vi "TestFlipper.vi"() -> ()   [LabVIEW 2020]
uses:
  C:/Program Files (x86)/Thorlabs/Kinesis/Thorlabs.MotionControl.FilterFlipperCLI.dll
  Program Files (x86)/Thorlabs/Kinesis/Thorlabs.MotionControl.FilterFlipperCLI.dll
  C:/Program Files (x86)/Thorlabs/Kinesis/Thorlabs.MotionControl.DeviceManagerCLI.dll
  Program Files (x86)/Thorlabs/Kinesis/Thorlabs.MotionControl.DeviceManagerCLI.dll
panel:
  in  "Postion":enum32{"NA", "Position1", "Position2"}(ring)
  in  "GET":bool
  in  "SET":bool
  in  "position":u32
  in  "INIT":bool
  out "Status array":bool[](array[boolean])
  in  "OK":bool
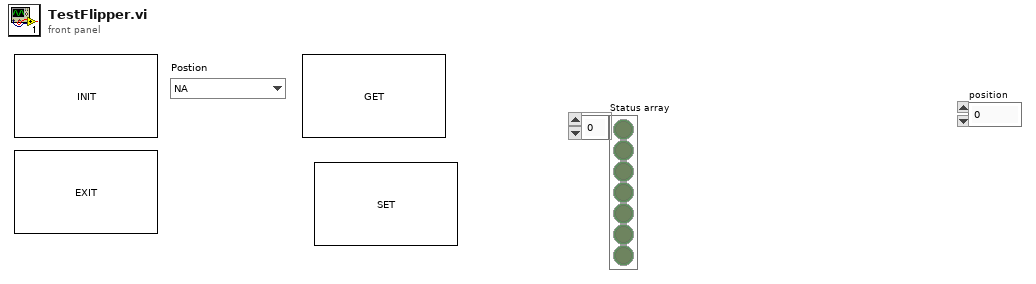
[diagram p1: front panel]
types:
  T1 = enum32{"Invalid", "Standard", "Closed", "Hidden", "Minimized", "Maximized"}
  T2 = enum32{"invalid app kind", "Development System", "Run Time System", "Student Edition", "Embedded LabVIEW", "Evaluation", "Custom"}
  T3 = cluster{"Core":cluster{"Current VI Reference":refnum<vi>, "Close Panel on Exit?":bool}, "Flipper":refnum<k24>, "Device":refnum<k24>}
  T4 = cluster{"Current VI Reference":refnum<vi>, "Close Panel on Exit?":bool}
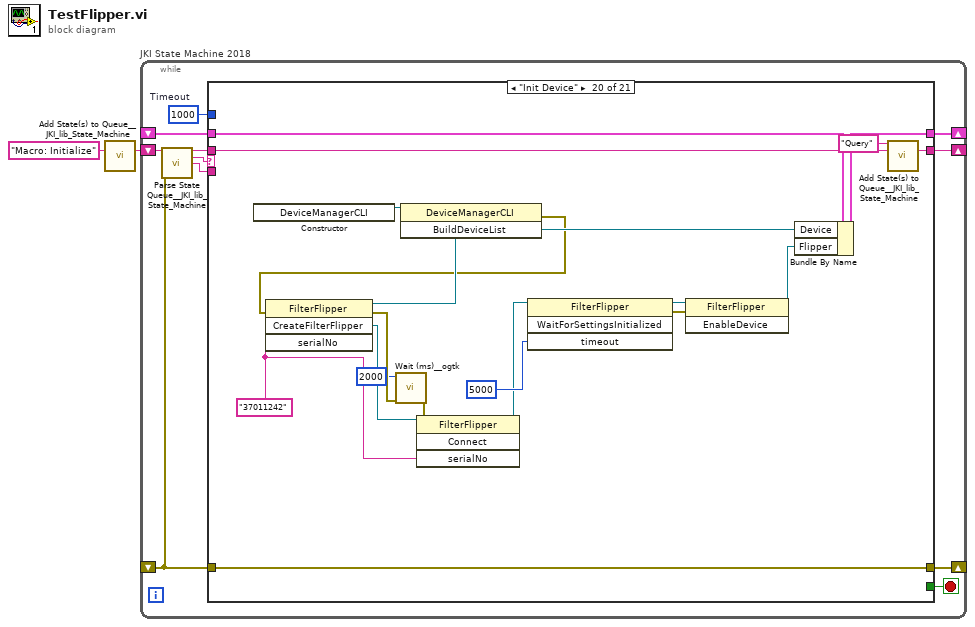
[diagram p0: block diagram]
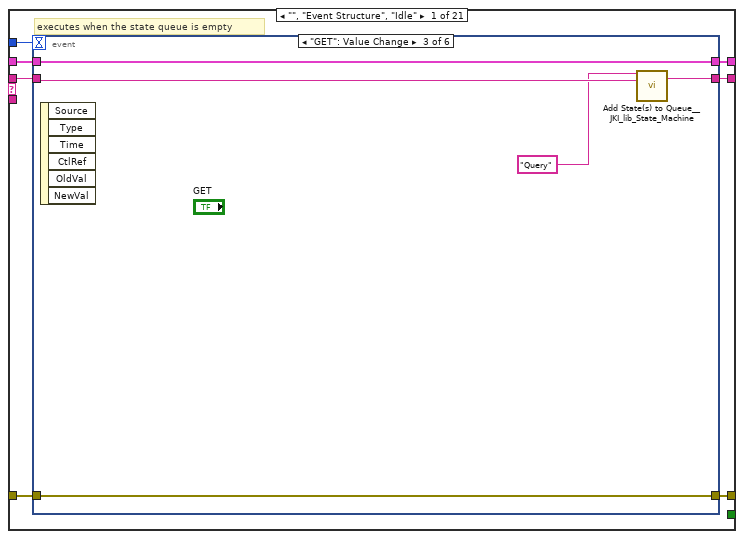
[diagram p2: hidden frame]
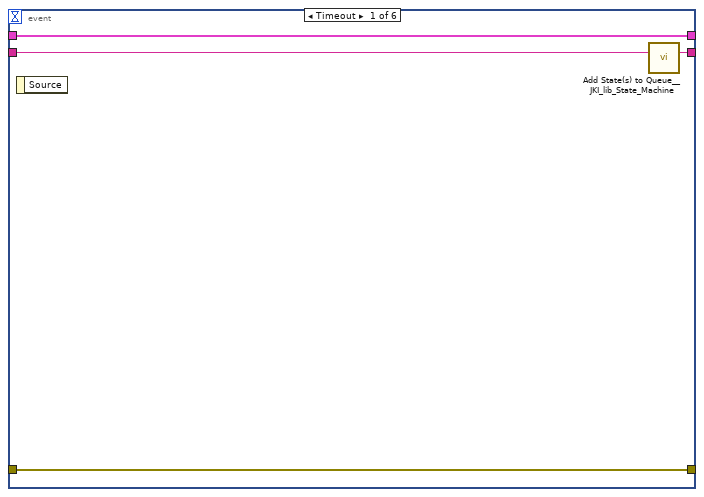
[diagram p3: hidden frame]
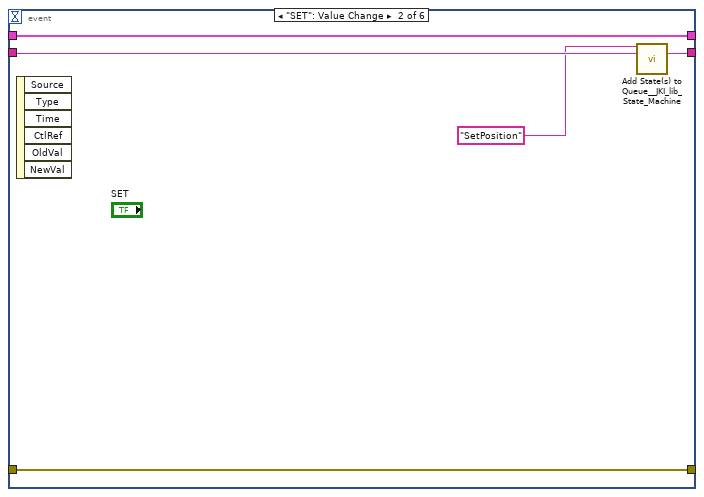
[diagram p4: hidden frame]
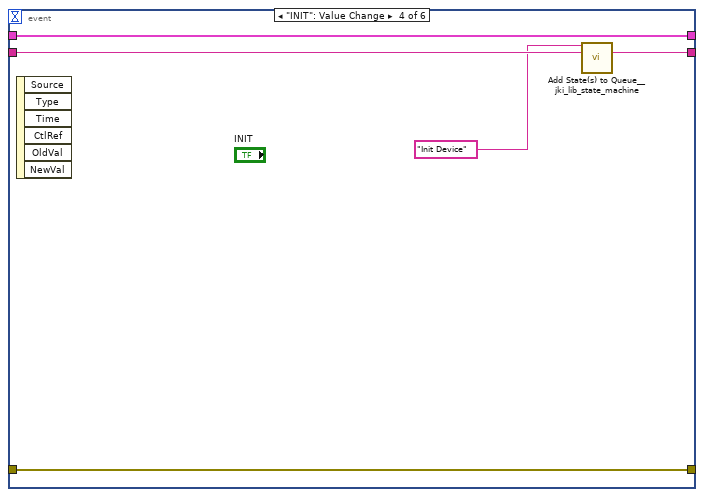
[diagram p5: hidden frame]
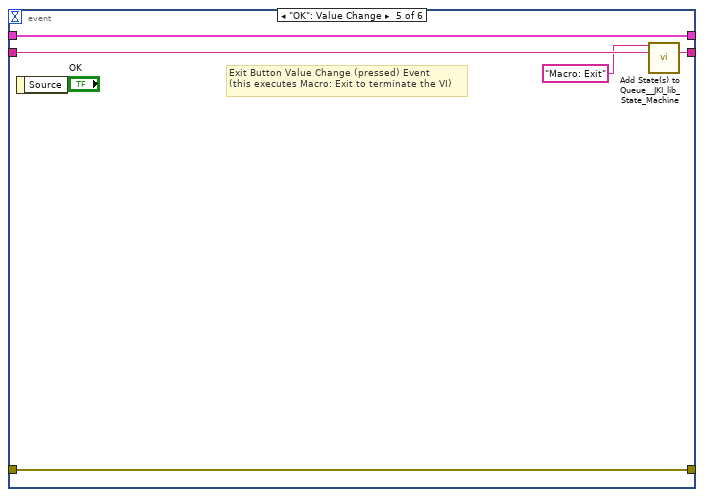
[diagram p6: hidden frame]
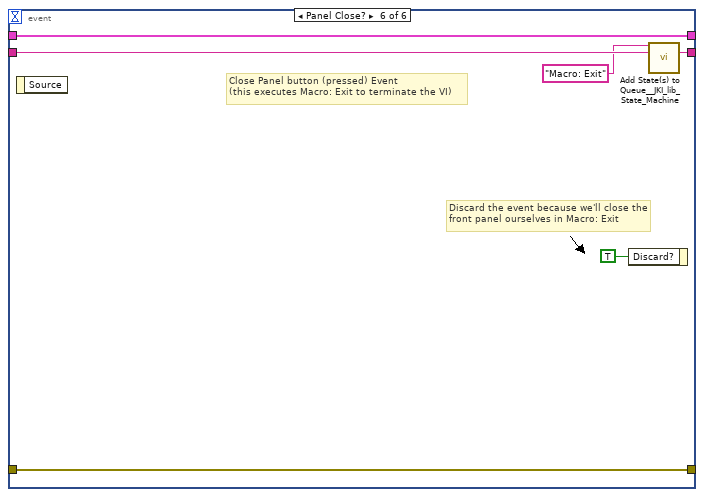
[diagram p7: hidden frame]
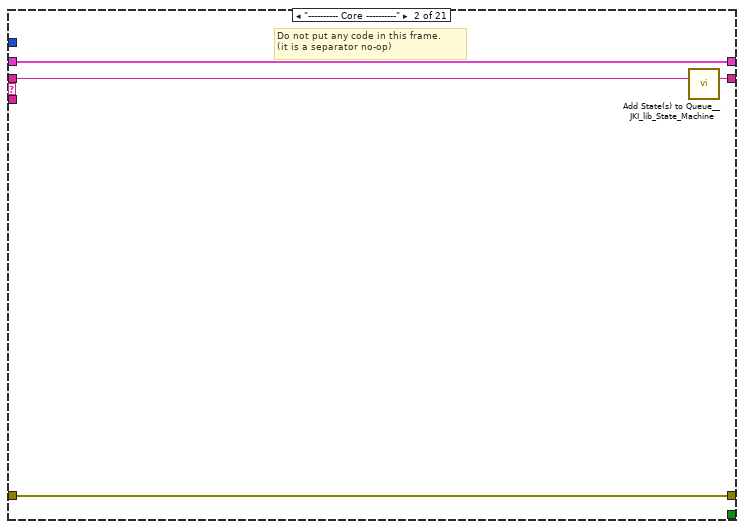
[diagram p8: hidden frame]
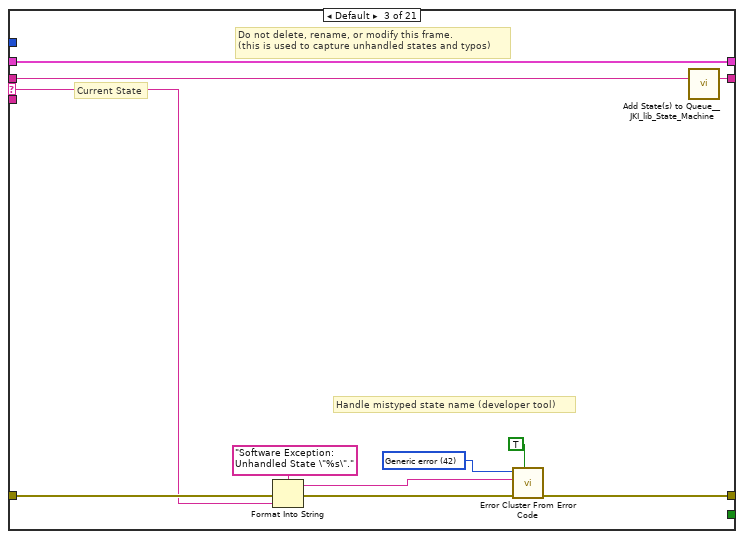
[diagram p9: hidden frame]
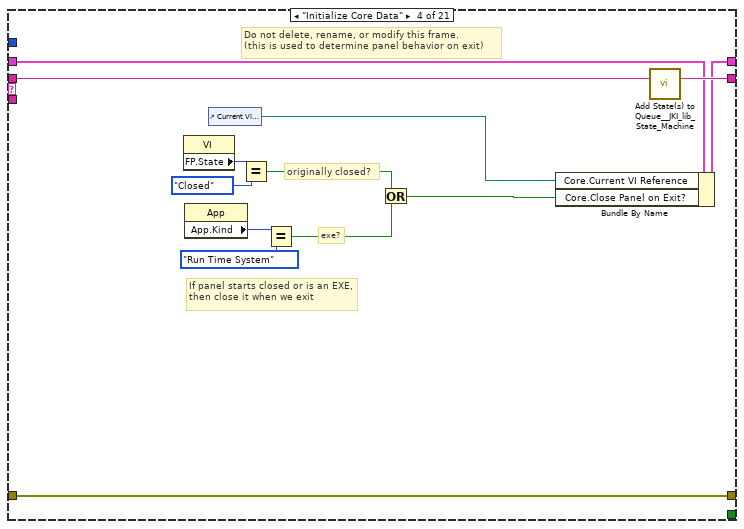
[diagram p10: hidden frame]
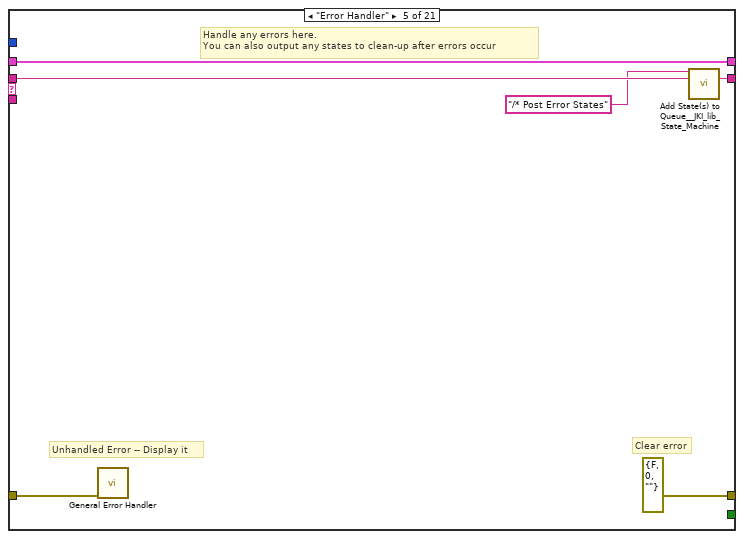
[diagram p11: hidden frame]
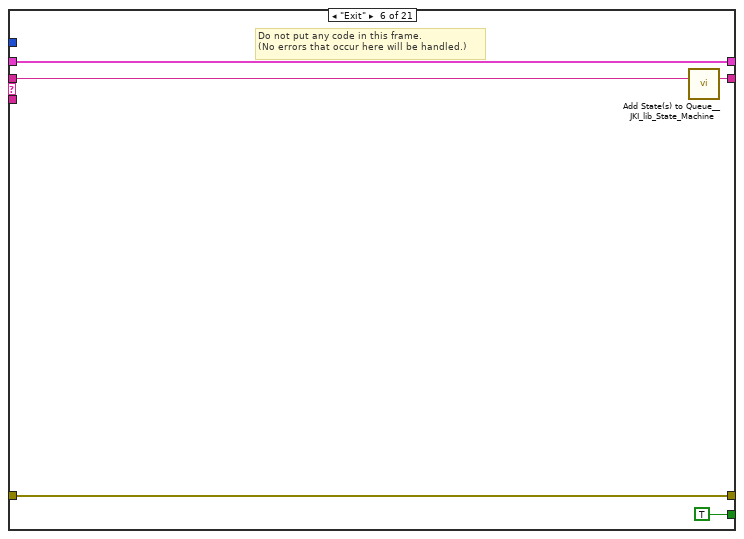
[diagram p12: hidden frame]
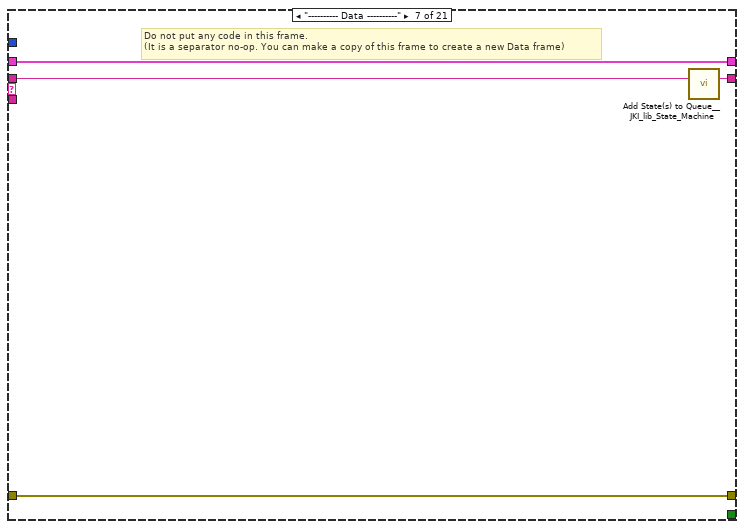
[diagram p13: hidden frame]
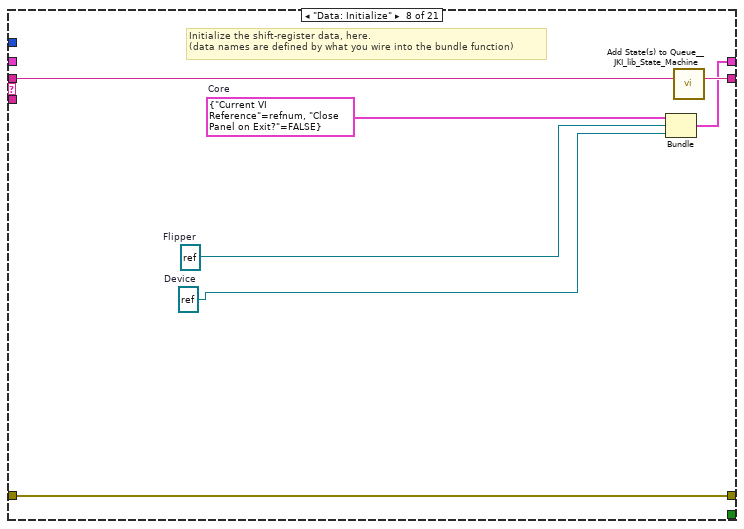
[diagram p14: hidden frame]
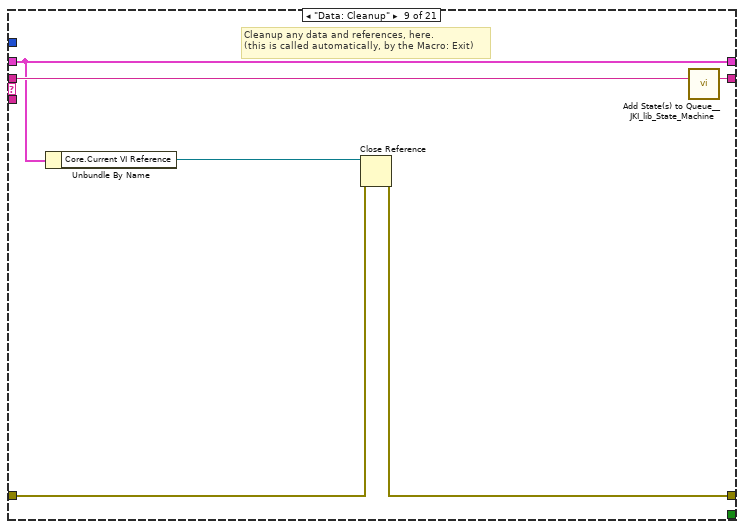
[diagram p15: hidden frame]
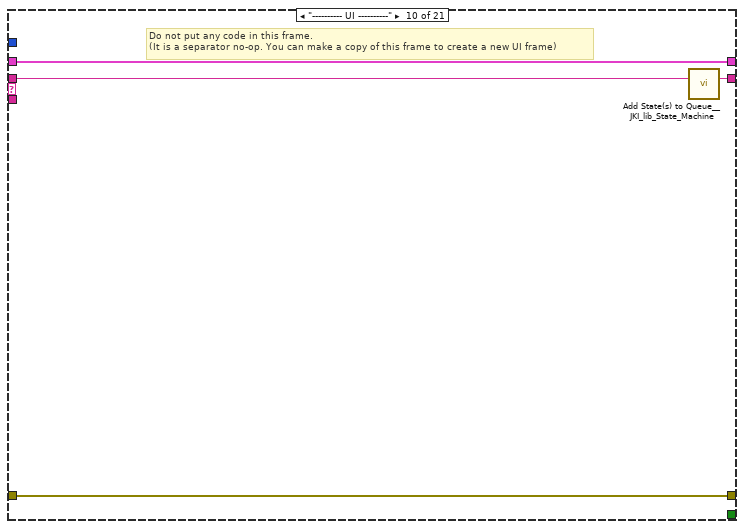
[diagram p16: hidden frame]
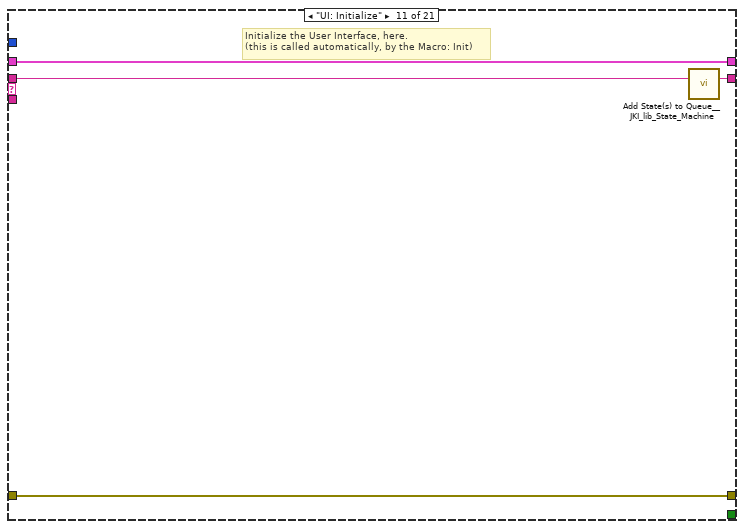
[diagram p17: hidden frame]
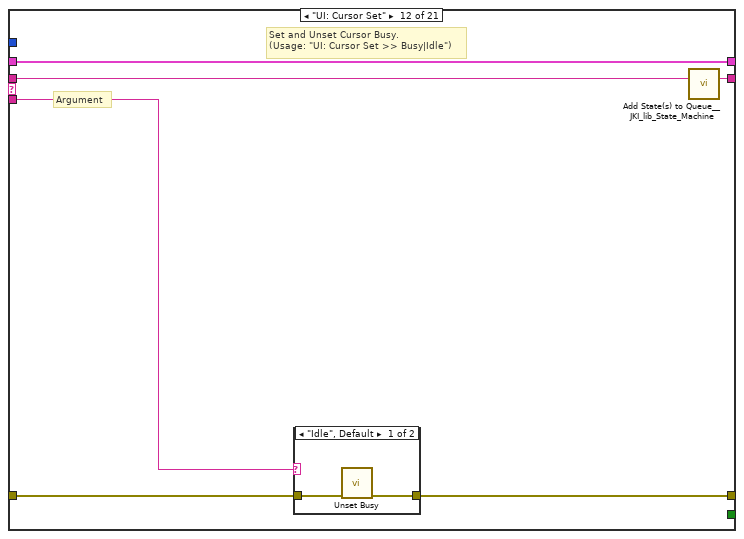
[diagram p18: hidden frame]
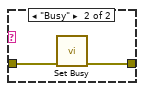
[diagram p19: hidden frame]
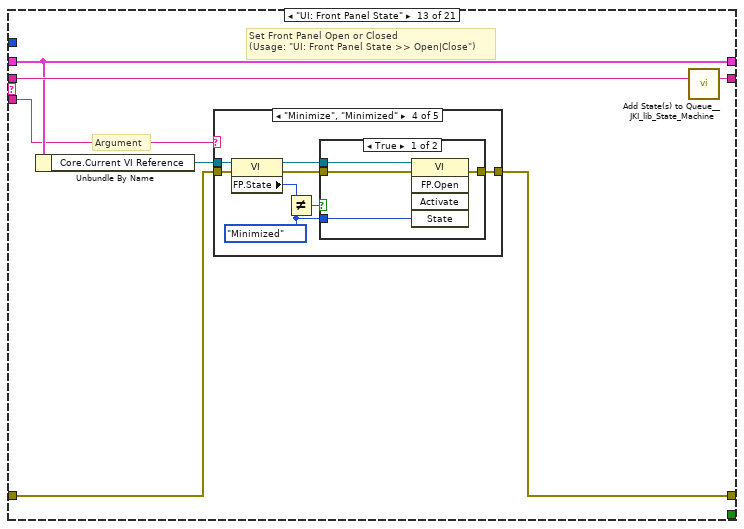
[diagram p20: hidden frame]
diagram:
  n1 = call <vilib>:"Add State(s) to Queue__JKI_lib_State_Machine.vi"("State(s) in (\"\")"="Macro: Initialize") -> ("States Out"=w2:string)  [unwired: 14 in]
  n2 = while "JKI State Machine 2018" {
    shift-right: [w6] -> _
    shift-left: _ -> [w5]
    shift-right: [w9] -> _
    shift-left: _ -> [w3]
    shift-right: [w8] -> _
    shift-left: w2 -> [w10]
    stop <- w7 stop-if-true
    w4 = 1000  # Timeout
    n3 = call <vilib>:"Parse State Queue__JKI_lib_State_Machine.vi"("State Queue"=w10, "Error In (no error)"=w3) -> ("Remaining States"=w12:string, "Current State"=w13:string, "Arguments"=w11:string)  [unwired: 11 in]
    n4 = case shown="\"Init Device\"" w13 {
      selector: w13 -> [_ _ w55 _ _ _ _ _ _ _ _ _ _ _ _ _ _ _ _ _ _]
      tunnel: w12 -> [w20 w54 w59 w78 w84 w89 w93 w100 w106 w110 w114 w120 w131 w200 w205 w215 w219 w235 w247 w266 w281]
      tunnel: w11 -> [_ _ _ _ _ _ _ _ _ _ _ w115 w125 _ _ _ _ _ _ _ _]
      tunnel: w5 -> [w18 w51 w57 w71 w81 w87 w90 _ w101 w107 w112 w118 w127 w197 w202 w212 w216 w233 w241 w263 w271]
      tunnel: [w17 w52 w61 w75 errorcluster {"status"=FALSE, "code"=0, "source"=""} ("error out") w86 w91 w97 w102 w108 w111 w116 w128 w198 w203 w213 w217 w221 w245 w264 w279] -> w9
      tunnel: w3 -> [w16 w52 w60 w75 w80 w86 w91 w97 w103 w108 w111 w117 w129 w198 w203 w213 w217 w229 w245 w264 w279]
      tunnel: [w19 w53 w58 w77 w83 w88 w92 w99 w105 w109 w113 w119 w130 w199 w204 w214 w218 w234 w246 w265 w280] -> w8
      tunnel: [_ _ _ _ _ TRUE _ _ _ _ _ _ _ _ _ _ _ _ _ _ _] -> w7
      tunnel: [w15 w51 w57 w76 w81 w87 w90 w98 w101 w107 w112 w118 w127 w197 w202 w212 w216 w230 w241 w259 w270] -> w6
      tunnel: w4 -> [w14 _ _ _ _ _ _ _ _ _ _ _ _ _ _ _ _ _ _ _ _]
      frame "", "Event Structure", "Idle" {
        # "executes when the state queue is empty"
        n5 = event shown="[2] \"GET\": Value Change" {
          selector: _ -> [_ _ _ _ _ _]
          dyn-events: _ -> [_ _ _ _ _ _]
          timeout: w14 -> [_ _ _ _ _ _]
          tunnel: w20 -> [w24 w26 w32 w37 w44 w50]
          tunnel: [w23 w27 w33 w36 w43 w49] -> w19
          tunnel: w18 -> [w21 w29 w34 w39 w41 w47]
          tunnel: [w22 w28 w30 w38 w42 w48] -> w17
          tunnel: w16 -> [w22 w28 w30 w38 w42 w48]
          tunnel: [w21 w29 w34 w39 w41 w47] -> w15
          event Timeout {
            n6 = event-data() -> ()  [unwired: 1 in, 1 out]
            n7 = call <vilib>:"Add State(s) to Queue__JKI_lib_State_Machine.vi"("State(s) in (\"\")"=w24) -> ("States Out"=w23:string)  [unwired: 14 in]
          }
          event "SET": Value Change {
            n8 = event-data() -> ()  [unwired: 1 in, 6 out]
            n9 = call <vilib>:"Add State(s) to Queue__JKI_lib_State_Machine.vi"("State(s) in Front (\"\")"="SetPosition" ("State(s) in Front (\"\")"), "State(s) in (\"\")"=w26) -> ("States Out"=w27:string)  [unwired: 13 in]
          }
          event "GET": Value Change {
            n10 = event-data() -> ()  [unwired: 1 in, 6 out]
            n11 = call <vilib>:"Add State(s) to Queue__JKI_lib_State_Machine.vi"("State(s) in Front (\"\")"="Query" ("State(s) in Front (\"\")"), "State(s) in (\"\")"=w32) -> ("States Out"=w33:string)  [unwired: 13 in]
          }
          event "INIT": Value Change {
            n12 = event-data() -> ()  [unwired: 1 in, 6 out]
            n13 = call <vilib>:"Add State(s) to Queue__jki_lib_state_machine.vi"("State(s) in Front (\"\")"="Init Device" ("State(s) in Front (\"\")"), "State(s) in (\"\")"=w37) -> ("States Out"=w36:string)  [unwired: 13 in]
          }
          event "OK": Value Change {
            # "Exit Button Value Change (pressed) Event\n(this executes Macro: Exit to terminate the VI)"
            n14 = event-data() -> ()  [unwired: 1 in, 1 out]
            n15 = call <vilib>:"Add State(s) to Queue__JKI_lib_State_Machine.vi"("State(s) in Front (\"\")"="Macro: Exit", "State(s) in (\"\")"=w44) -> ("States Out"=w43:string)  [unwired: 13 in]
          }
          event Panel Close? {
            # "Discard the event because we'll close the front panel ourselves in Macro: Exit"
            # "Close Panel button (pressed) Event\n(this executes Macro: Exit to terminate the VI)"
            n16 = event-data() -> ()  [unwired: 1 in, 1 out]
            n17 = event-data("Discard?"=TRUE) -> ()  [unwired: 1 in, 1 out]
            n18 = call <vilib>:"Add State(s) to Queue__JKI_lib_State_Machine.vi"("State(s) in Front (\"\")"="Macro: Exit", "State(s) in (\"\")"=w50) -> ("States Out"=w49:string)  [unwired: 13 in]
          }
        }
      }
      frame "---------- Core ----------" {
        # "Do not put any code in this frame.\n(it is a separator no-op)"
        n19 = call <vilib>:"Add State(s) to Queue__JKI_lib_State_Machine.vi"("State(s) in (\"\")"=w54) -> ("States Out"=w53:string)  [unwired: 14 in]
      }
      frame Default {
        w64 = 42 items=["No error", "Argument error", "Memory is full", "Out of zone", "End of file", "File already open", "Generic file I/O error", "File not found", "File permission error", "Disk is full", "Duplicate path", "Too many files open", "System feature not enabled", "Resource file not found", "Cannot add resource", "Resource not found", "Image not found", "Image memory error", "Pen does not exist", "Config type invalid", "Config token not found", "Config parse error", "Config memory error", "Bad external code format", "Bad external code offset", "External code not present", "Null window", "Destroy window error", "Null menu", "Print aborted", "Bad print record", "Print driver error", "Windows error during printing", "Memory error during printing", "Print dialog error", "Generic print error", "Invalid device refnum", "Device not found", "Device parameter error", "Device unit error", "Cannot open device", "Device call aborted", "Generic error", "Cancelled by user", "Object ID too low", "Object ID too high", "Object not in heap", "Unknown heap", "Unknown object (invalid DefProc)", "Unknown object (DefProc not in table)", "Message out of range", "Invalid (null) method", "Unknown message", "Manager call not supported", "Bad address", "Network operation in progress", "Network operation timed out", "Connection is busy", "Network attribute not supported", "Network error", "Address in use", "System out of memory", "Connection aborted", "Connection refused", "Not connected", "Already connected", "Connection closed", "Initialization error (interapplication manager)", "Bad occurrence", "Wait on unbound occurrence handler", "Occurrence queue overflow", "Datalog type conflict", "Unused", "Unrecognized type (interapplication manager)", "Memory corrupt", "Failed to make temporary DLL", "Old CIN version", "Drag socket not found", "Failed to load drop-object", "Failed to register OLE object", "Failed to release OLE object", "Format specifier type mismatch", "Unknown format specifier", "Too few format specifiers", "Too many format specifiers", "Scan failed", "Newer CIN version", "Error converting to variant", "Runtime menu error", "Password tampered", "Variant attribute not found", "Incompatible variant data type", "Event data is not available", "Event Store is not present", "Occurrence is not found", "Event Queue is not created", "Event info is not available", "Refnum passed is NULL", "Error retrieving Class GUID", "Error retrieving CoClass GUID", "Error retrieving TypeLib GUID.", "Bad built application magic bytes.", "Specific driver is different from the specific driver associated with the Logical Name.", "There is no session opened to the class driver.", "Max Error", "MAX - Error with config objects", "MAX - Error loading configuration", "MAX - Group not supported"]
        # "Current State"
        # "Do not delete, rename, or modify this frame.\n(this is used to capture unhandled states and typos)"
        # "Handle mistyped state name (developer tool)"
        n20 = Format Into String(format string="Software Exception: Unhandled State \"%s\"." ("message"), error in=w60, w55) -> (resulting string=w63:string, error out=w62:errorcluster)  [unwired: 1 in]
        n21 = call <vilib>:"Error Cluster From Error Code.vi"("show call chain? (False)"=TRUE, "error in (no error)"=w62, "error message (\"\")"=w63, "error code (0)"=w64) -> ("error out"=w61:errorcluster)  [unwired: 5 in]
        n22 = call <vilib>:"Add State(s) to Queue__JKI_lib_State_Machine.vi"("State(s) in (\"\")"=w59) -> ("States Out"=w58:string)  [unwired: 14 in]
      }
      frame "Initialize Core Data" {
        # "Do not delete, rename, or modify this frame.\n(this is used to determine panel behavior on exit)"
        # "originally closed?"
        # "exe?"
        # "If panel starts closed or is an EXE, then close it when we exit"
        n23 = property class="VI"() -> ("FP.State"=w68:T1)  [unwired: 2 in, 2 out]
        n24 = property class="App"() -> ("App.Kind"=w74:T2)  [unwired: 2 in, 2 out]
        n25 = control-ref of="Current VI Reference"() -> (w69:refnum<vi>)
        n26 = Equal?(x=w68, y=T1."Closed" ("Front Panel Window:State")) -> (x = y?=w66:bool)
        n27 = Equal?(x=w74, y=T2."Run Time System" ("Application:Kind")) -> (x = y?=w72:bool)
        n28 = Or(x=w66, y=w72) -> (x .or. y?=w70:bool)
        n29 = Bundle By Name(cluster=w71, "Core.Current VI Reference"=w69, "Core.Close Panel on Exit?"=w70) -> (w76:T3)
        n30 = call <vilib>:"Add State(s) to Queue__JKI_lib_State_Machine.vi"("State(s) in (\"\")"=w78) -> ("States Out"=w77:string)  [unwired: 14 in]
      }
      frame "Error Handler" {
        # "Unhandled Error -- Display it"
        # "Handle any errors here.\nYou can also output any states to clean-up after errors occur"
        # "Clear error"
        n31 = call <vilib>:"General Error Handler.vi"("error in (no error)"=w80) -> ()  [unwired: 10 in, 5 out]
        n32 = call <vilib>:"Add State(s) to Queue__JKI_lib_State_Machine.vi"("State(s) in Front (\"\")"="/* Post Error States", "State(s) in (\"\")"=w84) -> ("States Out"=w83:string)  [unwired: 13 in]
      }
      frame "Exit" {
        # "Do not put any code in this frame.\n(No errors that occur here will be handled.)"
        n33 = call <vilib>:"Add State(s) to Queue__JKI_lib_State_Machine.vi"("State(s) in (\"\")"=w89) -> ("States Out"=w88:string)  [unwired: 14 in]
      }
      frame "---------- Data ----------" {
        # "Do not put any code in this frame.\n(It is a separator no-op. You can make a copy of this frame to create a new Data frame)"
        n34 = call <vilib>:"Add State(s) to Queue__JKI_lib_State_Machine.vi"("State(s) in (\"\")"=w93) -> ("States Out"=w92:string)  [unwired: 14 in]
      }
      frame "Data: Initialize" {
        w94 = refnum<k24> refnum  # Device
        w95 = refnum<k24> refnum  # Flipper
        w96 = T4 {"Current VI Reference"=refnum, "Close Panel on Exit?"=FALSE}  # Core
        # "Initialize the shift-register data, here.\n(data names are defined by what you wire into the bundle function)"
        n35 = Bundle("Core"=w96, "Flipper"=w95, "Device"=w94) -> (w98:T3)  [unwired: 1 in]
        n36 = call <vilib>:"Add State(s) to Queue__JKI_lib_State_Machine.vi"("State(s) in (\"\")"=w100) -> ("States Out"=w99:string)  [unwired: 14 in]
      }
      frame "Data: Cleanup" {
        # "Cleanup any data and references, here.\n(this is called automatically, by the Macro: Exit)"
        n37 = Unbundle By Name(w101) -> ("Core.Current VI Reference"=w104:refnum<vi>)
        n38 = Close Reference(reference=w104, error in (no error)=w103) -> (error out=w102:errorcluster)
        n39 = call <vilib>:"Add State(s) to Queue__JKI_lib_State_Machine.vi"("State(s) in (\"\")"=w106) -> ("States Out"=w105:string)  [unwired: 14 in]
      }
      frame "---------- UI ----------" {
        # "Do not put any code in this frame.\n(It is a separator no-op. You can make a copy of this frame to create a new UI frame)"
        n40 = call <vilib>:"Add State(s) to Queue__JKI_lib_State_Machine.vi"("State(s) in (\"\")"=w110) -> ("States Out"=w109:string)  [unwired: 14 in]
      }
      frame "UI: Initialize" {
        # "Initialize the User Interface, here.\n(this is called automatically, by the Macro: Init)"
        n41 = call <vilib>:"Add State(s) to Queue__JKI_lib_State_Machine.vi"("State(s) in (\"\")"=w114) -> ("States Out"=w113:string)  [unwired: 14 in]
      }
      frame "UI: Cursor Set" {
        # "Argument"
        # "Set and Unset Cursor Busy.\n(Usage: \"UI: Cursor Set >> Busy|Idle\")"
        n42 = case shown="\"Idle\", Default" w115 {
          tunnel: w117 -> [w122 w124]
          tunnel: [w121 w123] -> w116
          frame "Idle", Default {
            n43 = call <vilib>:"Unset Busy.vi"("error in (no error)"=w122) -> ("error out"=w121:errorcluster)  [unwired: 10 in]
          }
          frame "Busy" {
            n44 = call <vilib>:"Set Busy.vi"("error in (no error)"=w124) -> ("error out"=w123:errorcluster)  [unwired: 9 in, 1 out]
          }
        }
        n45 = call <vilib>:"Add State(s) to Queue__JKI_lib_State_Machine.vi"("State(s) in (\"\")"=w120) -> ("States Out"=w119:string)  [unwired: 14 in]
      }
      frame "UI: Front Panel State" {
        # "Argument"
        # "Set Front Panel Open or Closed\n(Usage: \"UI: Front Panel State >> Open|Close\")"
        n46 = Unbundle By Name(w127) -> ("Core.Current VI Reference"=w126:refnum<vi>)
        n47 = case shown="\"Minimize\", \"Minimized\"" w125 {
          tunnel: w129 -> [w137 w152 w163 w176 w189]
          tunnel: [w139 w153 w165 w178 w191] -> w128
          tunnel: w126 -> [w138 w150 w164 w177 w190]
          frame "Open", "Standard", Default {
            w132 = T1."Standard" ("State")
            n48 = property class="VI"(reference=w138, error in=w137) -> (reference out=w135:refnum<vi>, error out=w136:errorcluster, "FP.State"=w134:T1)
            n49 = Not Equal?(x=w134, y=w132) -> (x != y?=w133:bool)
            n50 = case shown="True" w133 {
              tunnel: [w143 w145] -> w139
              tunnel: w136 -> [w142 w145]
              tunnel: w135 -> [w141 _]
              tunnel: w132 -> [w140 _]
              frame True {
                n51 = invoke class="VI" method="FP.Open"(reference=w141, error in=w142, "Activate"=TRUE, "State"=w140) -> (error out=w143:errorcluster)  [unwired: 1 in, 4 out]
              }
              frame False {
              }
            }
          }
          frame "Close", "Closed" {
            n52 = property class="VI"(reference=w150, error in=w152) -> (reference out=w149:refnum<vi>, error out=w151:errorcluster, "FP.State"=w147:T1)
            n53 = Not Equal?(x=w147, y=T1."Closed" ("Front Panel Window:State")) -> (x != y?=w146:bool)
            n54 = case shown="True" w146 {
              tunnel: [w154 w157] -> w153
              tunnel: w151 -> [w154 w156]
              tunnel: w149 -> [_ w155]
              frame False {
              }
              frame True {
                n55 = invoke class="VI" method="FP.Close"(reference=w155, error in=w156) -> (error out=w157:errorcluster)  [unwired: 1 in, 2 out]
              }
            }
          }
          frame "Hidden", "Hide" {
            w158 = T1."Hidden" ("State")
            n56 = property class="VI"(reference=w164, error in=w163) -> (reference out=w161:refnum<vi>, error out=w162:errorcluster, "FP.State"=w160:T1)
            n57 = Not Equal?(x=w160, y=w158) -> (x != y?=w159:bool)
            n58 = case shown="True" w159 {
              tunnel: [w169 w170] -> w165
              tunnel: w162 -> [w168 w170]
              tunnel: w161 -> [w167 _]
              tunnel: w158 -> [w166 _]
              frame True {
                n59 = invoke class="VI" method="FP.Open"(reference=w167, error in=w168, "State"=w166) -> (error out=w169:errorcluster)  [unwired: 2 in, 4 out]
              }
              frame False {
              }
            }
          }
          frame "Minimize", "Minimized" {
            w171 = T1."Minimized" ("State")
            n60 = property class="VI"(reference=w177, error in=w176) -> (reference out=w174:refnum<vi>, error out=w175:errorcluster, "FP.State"=w173:T1)
            n61 = Not Equal?(x=w173, y=w171) -> (x != y?=w172:bool)
            n62 = case shown="True" w172 {
              tunnel: [w182 w183] -> w178
              tunnel: w175 -> [w181 w183]
              tunnel: w174 -> [w180 _]
              tunnel: w171 -> [w179 _]
              frame True {
                n63 = invoke class="VI" method="FP.Open"(reference=w180, error in=w181, "State"=w179) -> (error out=w182:errorcluster)  [unwired: 2 in, 4 out]
              }
              frame False {
              }
            }
          }
          frame "Maximize", "Maximized" {
            w184 = T1."Maximized" ("State")
            n64 = property class="VI"(reference=w190, error in=w189) -> (reference out=w187:refnum<vi>, error out=w188:errorcluster, "FP.State"=w186:T1)
            n65 = Not Equal?(x=w186, y=w184) -> (x != y?=w185:bool)
            n66 = case shown="True" w185 {
              tunnel: [w195 w196] -> w191
              tunnel: w188 -> [w194 w196]
              tunnel: w187 -> [w193 _]
              tunnel: w184 -> [w192 _]
              frame True {
                n67 = invoke class="VI" method="FP.Open"(reference=w193, error in=w194, "State"=w192) -> (error out=w195:errorcluster)  [unwired: 2 in, 4 out]
              }
              frame False {
              }
            }
          }
        }
        n68 = call <vilib>:"Add State(s) to Queue__JKI_lib_State_Machine.vi"("State(s) in (\"\")"=w131) -> ("States Out"=w130:string)  [unwired: 14 in]
      }
      frame "---------- Macro ----------" {
        # "Do not put any code in this frame.\n(It is a separator no-op. You can make a copy of this frame to create a new Macro frame)"
        n69 = call <vilib>:"Add State(s) to Queue__JKI_lib_State_Machine.vi"("State(s) in (\"\")"=w200) -> ("States Out"=w199:string)  [unwired: 14 in]
      }
      frame "Macro: Initialize" {
        w201 = "Data: Initialize\nInitialize Core Data\nUI: Initialize\nUI: Front Panel State >> Open"  # Data: Initialize Initialize Core Data UI: Initialize UI: Front Panel State >> Open
        # "Initialization Macro\n(This is called once, when the VI starts)"
        n70 = call <vilib>:"Add State(s) to Queue__JKI_lib_State_Machine.vi"("State(s) in Front (\"\")"=w201, "State(s) in (\"\")"=w205) -> ("States Out"=w204:string)  [unwired: 13 in]
      }
      frame "Macro: Exit" {
        # "Exit Macro\n(This is called once, when the VI exits)"
        n71 = Unbundle By Name(w212) -> ("Core.Close Panel on Exit?"=w211:bool)
        n72 = Select(t="UI: Front Panel State >> Close", s=w211, f="") -> (s? t:f=w208:string)
        n73 = call <vilib>:"Add State(s) to Queue__JKI_lib_State_Machine.vi"("State(s) in (\"\")"=w208, "State(s) at Back (\"\")"="DIsconnnect\nData: Cleanup\nExit") -> ("States Out"=w206:string)  [unwired: 13 in]
        n74 = call <vilib>:"Add State(s) to Queue__JKI_lib_State_Machine.vi"("State(s) in Front (\"\")"=w206, "State(s) in (\"\")"=w215) -> ("States Out"=w214:string)  [unwired: 13 in]
      }
      frame "---------- New Category ----------" {
        # "Template Separator\n(You can make a copy of, or modify, this frame)"
        n75 = call <vilib>:"Add State(s) to Queue__JKI_lib_State_Machine.vi"("State(s) in (\"\")"=w219) -> ("States Out"=w218:string)  [unwired: 14 in]
      }
      frame "SetPosition" {
        n76 = Unbundle By Name(w233) -> ("Flipper"=w228:refnum<k24>)
        n77 = invoke class="FilterFlipper" method="ClearDeviceExceptions"(reference=w228) -> (reference out=w227:refnum<k24>)  [unwired: 2 in, 2 out]
        n78 = invoke class="FilterFlipper" method="SetPosition"(reference=w227, error in=w229, "position"="Postion", "waitTimeout"=2000) -> (reference out=w224:refnum<k24>, error out=w226:errorcluster)  [unwired: 1 in, 3 out]
        n79 = call <userlib>:"Wait (ms)__ogtk.vi"("error in (no error)"=w226, "milliseconds to wait"=u32 50) -> ("error out"=w222:errorcluster)  [unwired: 8 in, 1 out]
        n80 = Unbundle By Name(w222) -> ("code"=w223:i32)
        n81 = case shown="0, Default" w223 {
          tunnel: [w236 errorcluster {"status"=FALSE, "code"=0, "source"=""} ("error out")] -> w221
          tunnel: w222 -> [w236 _]
          frame 0, Default {
          }
          frame 1172 {
          }
        }
        n82 = Bundle By Name(cluster=w233, "Flipper"=w224) -> (w230:T3)
        n83 = call <vilib>:"Add State(s) to Queue__JKI_lib_State_Machine.vi"("State(s) in Front (\"\")"="Query" ("State(s) in Front (\"\")"), "State(s) in (\"\")"=w235) -> ("States Out"=w234:string)  [unwired: 13 in]
      }
      frame "DIsconnnect" {
        # "Template Separator\n(You can make a copy of, or modify, this frame)"
        n84 = Unbundle By Name(w241) -> ("Device"=w238:refnum<k24>, "Flipper"=w244:refnum<k24>)
        n85 = invoke class="FilterFlipper" method="DisableDevice"(reference=w244) -> (reference out=w243:refnum<k24>, error out=w242:errorcluster)  [unwired: 2 in, 1 out]
        n86 = invoke class="FilterFlipper" method="Disconnect"(reference=w243, error in=w242) -> (reference out=w240:refnum<k24>, error out=w239:errorcluster)  [unwired: 1 in, 1 out]
        n87 = Close Reference(reference=w240, error in (no error)=w239) -> ()  [unwired: 1 out]
        n88 = Close Reference(reference=w238) -> ()  [unwired: 1 in, 1 out]
        n89 = call <vilib>:"Add State(s) to Queue__JKI_lib_State_Machine.vi"("State(s) in (\"\")"=w247) -> ("States Out"=w246:string)  [unwired: 14 in]
      }
      frame "Init Device" {
        w256 = "37011242" ("serialNo")
        n90 = constructor class="DeviceManagerCLI"() -> (reference out=w250:refnum<k24>)  [unwired: 3 in, 2 out]
        n91 = invoke class="DeviceManagerCLI" method="BuildDeviceList"(reference=w250) -> (error out=w249:errorcluster)  [unwired: 2 in, 2 out]
        n92 = invoke class="FilterFlipper" method="CreateFilterFlipper"(error in=w249, "serialNo"=w256) -> (reference out=w254:refnum<k24>, error out=w253:errorcluster, "CreateFilterFlipper"=w257:refnum<k24>)  [unwired: 2 in, 1 out]
        n93 = call <userlib>:"Wait (ms)__ogtk.vi"("error in (no error)"=w253, "milliseconds to wait"=u32 2000) -> ("error out"=w252:errorcluster)  [unwired: 8 in, 1 out]
        n94 = invoke class="FilterFlipper" method="Connect"(reference=w257, error in=w252, "serialNo"=w256) -> (reference out=w255:refnum<k24>)  [unwired: 1 in, 3 out]
        n95 = invoke class="FilterFlipper" method="WaitForSettingsInitialized"(reference=w255, "timeout"=5000) -> (reference out=w262:refnum<k24>, error out=w260:errorcluster)  [unwired: 2 in, 2 out]
        n96 = invoke class="FilterFlipper" method="EnableDevice"(reference=w262, error in=w260) -> (reference out=w258:refnum<k24>)  [unwired: 1 in, 2 out]
        n97 = Bundle By Name(cluster=w263, "Device"=w254, "Flipper"=w258) -> (w259:T3)
        n98 = call <vilib>:"Add State(s) to Queue__JKI_lib_State_Machine.vi"("State(s) in Front (\"\")"="Query" ("State(s) in Front (\"\")"), "State(s) in (\"\")"=w266) -> ("States Out"=w265:string)  [unwired: 13 in]
      }
      frame "Query" {
        (unwired) 500 ("waitTimeout")
        n99 = Unbundle By Name(w271) -> ("Flipper"=w278:refnum<k24>)
        n100 = invoke class="FilterFlipper" method="RequestStatus"(reference=w278) -> (reference out=w277:refnum<k24>, error out=w276:errorcluster)  [unwired: 2 in, 1 out]
        n101 = call <userlib>:"Wait (ms)__ogtk.vi"("error in (no error)"=w276, "milliseconds to wait"=u32 500) -> ("error out"=w268:errorcluster)  [unwired: 8 in, 1 out]
        n102 = invoke class="FilterFlipper" method="ClearDeviceExceptions"(reference=w277, error in=w268) -> (reference out=w275:refnum<k24>, error out=w274:errorcluster)  [unwired: 1 in, 1 out]
        n103 = invoke class="FilterFlipper" method="GetStatusBits"(reference=w275, error in=w274) -> (reference out=w269:refnum<k24>, "GetStatusBits"=w273:u32)  [unwired: 1 in, 1 out]
        n104 = Number To Boolean Array(number=w273) -> (Boolean array=→"Status array":bool[])
        n105 = Bundle By Name(cluster=w271, "Flipper"=w269) -> (w270:T3)
        n106 = call <vilib>:"Add State(s) to Queue__JKI_lib_State_Machine.vi"("State(s) in (\"\")"=w281) -> ("States Out"=w280:string)  [unwired: 14 in]
      }
    }
  }
